vi "Regatron.G5.Rest Simple Example.vi"() -> ()   [LabVIEW 2021, in "G5 Regatron Custom Device Shared.lvlib"]
doc: "Simple Example to control a G5 device"
uses:
  G5 Regatron Custom Device/Shared/G5 Regatron Custom Device Shared.lvlib
  Regatron.G5.Rest System.llb/G5.Rest System Output References.ctl
  Regatron.G5.Rest System.llb/G5.Rest System Output Limits.ctl
  Regatron.G5.Rest System.llb/G5.Rest System Output Values.ctl
  Regatron.G5.Rest Handle.llb/G5.Rest Status.ctl
  Regatron.G5.Rest System.llb/G5.Rest System Output Limits Datasource.ctl
  Regatron.G5.Rest System.llb/G5.Rest System Output References Datasource.ctl
  Regatron.G5.Rest System.llb/G5.Rest System Clear Inicidents.ctl
  Regatron.G5.Rest.lvlib
panel:
  in  "Registerkartenelement":enum32{"Power", "Limits"}(tab)
  in  "SET Output Control":T1(ring)
  out "Output Values":T2 {"Power W" format="%#.2f"; "Load R Ohm" format="%#_3e"; "Power kW" format="%#_3e"; "Current A" format="%#.2f"; "Voltage V" format="%#.2f"}
  in  "Clear Error & Warnings":bool
  out "State":T3(ring)=enum."Ready"
  in  "Power OFF/ON":bool
  in  "SET Output Reference":T4 {"Load R Ohm" format="%#_3e"; "Power W" format="%#.2f"; "Current A" format="%#.2f"; "Voltage V" format="%#.2f"}
  out "Device found":bool
  out "System Device":i32
  in  "SET Output Limit":T5 {"Power Lower Limit W" format="%#.2f"; "Power Upper Limit W" format="%#.2f"; "Current Lower Limit A" format="%#.2f"; "Current Upper Limit A" format="%#.2f"; "Voltage Lower Limit V" format="%#.2f"; "Voltage Upper Limit V" format="%#.2f"}
  in  "Stopp-Schaltfläche":bool
  out "Error Out":errorcluster
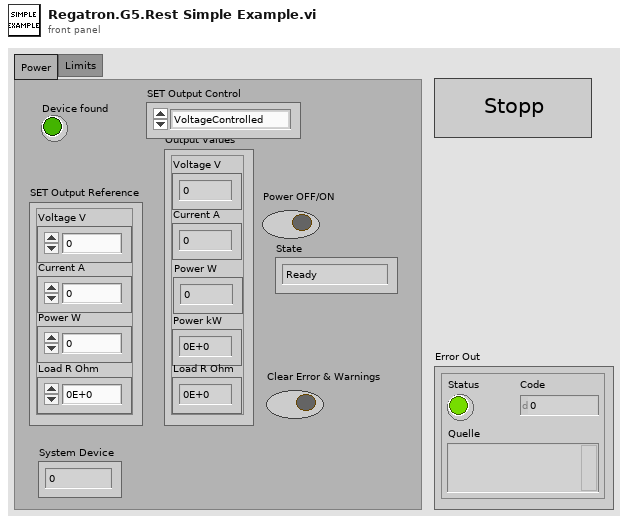
[diagram p1: front panel]
types:
  T1 = enum16{"VoltageControlled", "CurrentControlled", "PowerControlled", "ResistanceControlled"}
  T2 = typedef "G5 Regatron Custom Device Shared.lvlib/Regatron.G5.Rest.lvlib/G5.Rest System Output Values.ctl" = cluster{"Voltage V":sgl, "Current A":sgl, "Power W":sgl, "Power kW":sgl, "Load R Ohm":sgl}
  T3 = enum16{"Undefined", "PowerUp", "NotReady", "Ready", "VoltageOnPrepare", "VoltageOn", "VoltageOnLeave", "Test", "FirmwareUpdate"}
  T4 = typedef "G5 Regatron Custom Device Shared.lvlib/Regatron.G5.Rest.lvlib/G5.Rest System Output References.ctl" = cluster{"Voltage V":sgl, "Current A":sgl, "Power W":sgl, "Load R Ohm":sgl}
  T5 = typedef "G5 Regatron Custom Device Shared.lvlib/Regatron.G5.Rest.lvlib/G5.Rest System Output Limits.ctl" = cluster{"Voltage Upper Limit V":sgl, "Voltage Lower Limit V":sgl, "Current Upper Limit A":sgl, "Current Lower Limit A":sgl, "Power Upper Limit W":sgl, "Power Lower Limit W":sgl}
  T6 = typedef "G5 Regatron Custom Device Shared.lvlib/Regatron.G5.Rest.lvlib/G5.Rest Status.ctl" = enum16{"Read", "Write"}
  T7 = typedef "G5 Regatron Custom Device Shared.lvlib/Regatron.G5.Rest.lvlib/G5.Rest System Clear Inicidents.ctl" = enum16{"Clear Errors and Warnings", "Clear Warnings", "Clear Errors"}
  T8 = typedef "G5 Regatron Custom Device Shared.lvlib/Regatron.G5.Rest.lvlib/G5.Rest System Output References Datasource.ctl" = enum16{"Voltage", "Current", "Power", "Load Resistance", "ALL"}[]
  T9 = typedef "G5 Regatron Custom Device Shared.lvlib/Regatron.G5.Rest.lvlib/G5.Rest System Output Limits Datasource.ctl" = enum16{"Voltage Upper Limit", "Voltage Lower Limit", "Current Upper Limit", "Current Lower Limit", "Power Upper Limit", "Power Lower Limit", "ALL"}[]
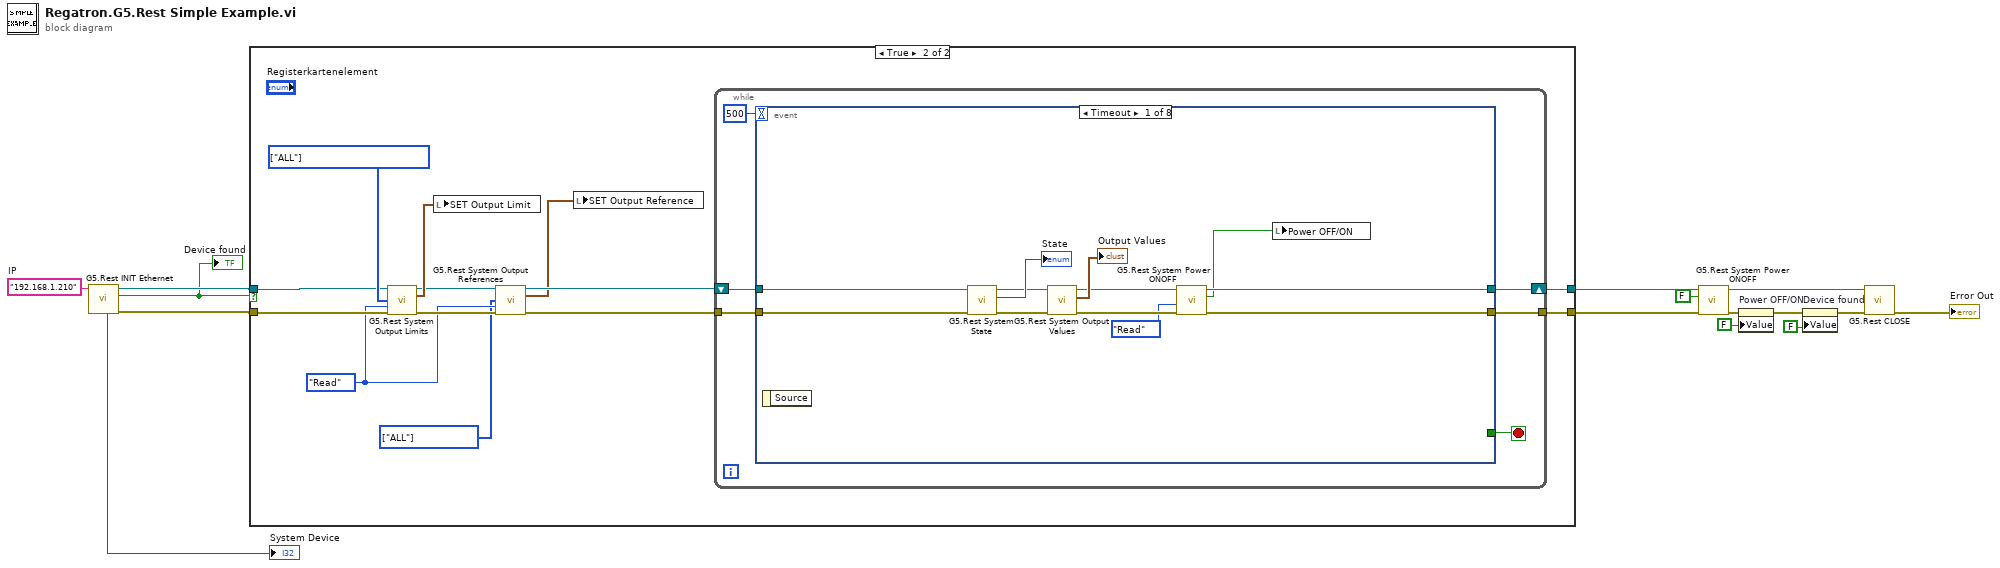
[diagram p0: block diagram]
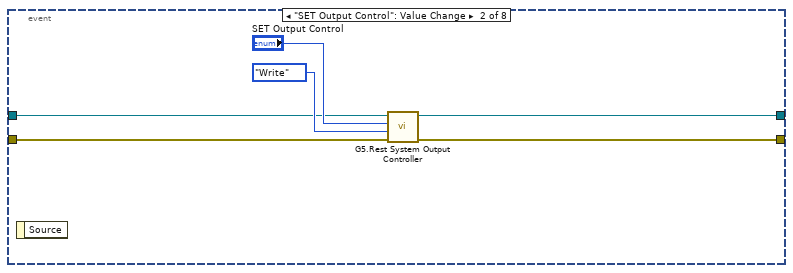
[diagram p3: hidden frame]
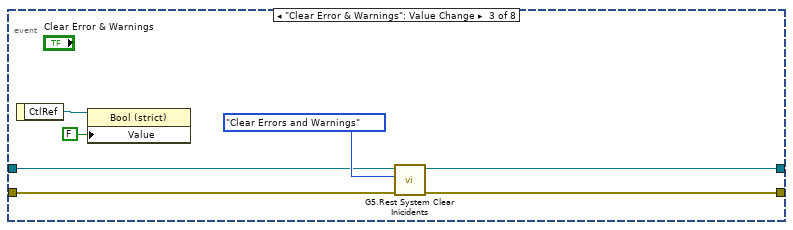
[diagram p4: hidden frame]
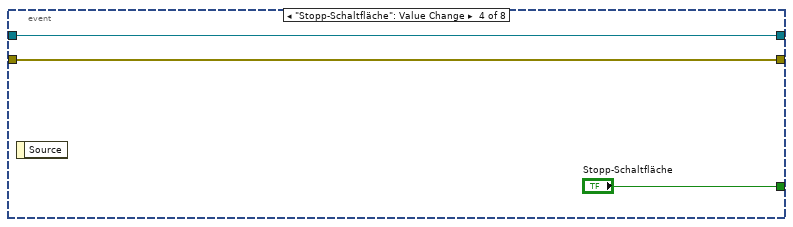
[diagram p5: hidden frame]
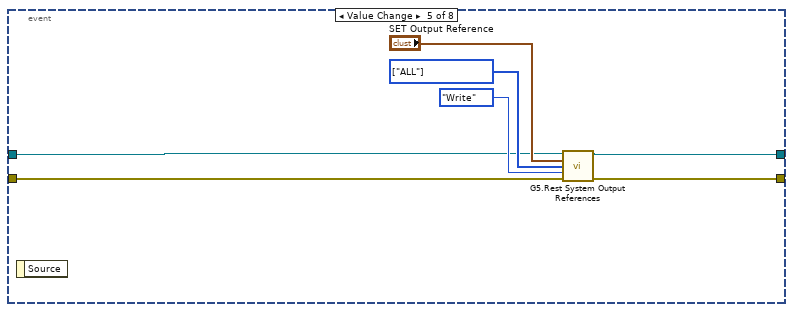
[diagram p6: hidden frame]
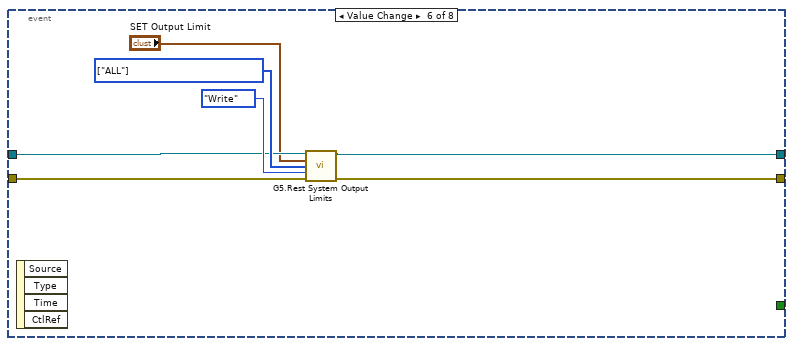
[diagram p7: hidden frame]
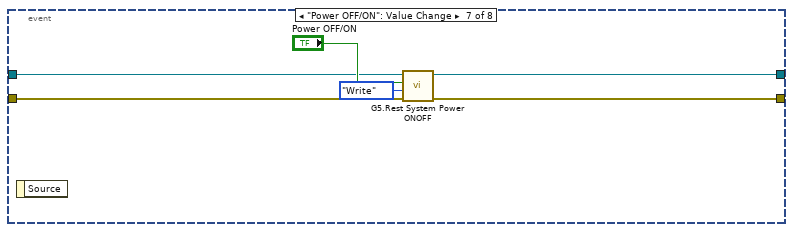
[diagram p8: hidden frame]
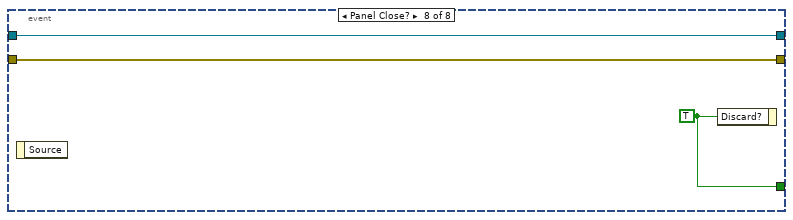
[diagram p9: hidden frame]
diagram:
  w5 = "192.168.1.210"  # IP
  n1 = call "G5.Rest INIT Ethernet.vi"("IP"=w5) -> ("error out"=w4:errorcluster, "Device found"=w2:bool, "G5 WEB API"=w3:refnum<class "REST Client.lvclass">, "Modul size"=→"System Device":i32)  [unwired: 6 in, 1 out]
  "Device found" <- w2
  n2 = case shown="True" w2 {
    tunnel: w4 -> [w17 w27]
    tunnel: [w17 w30] -> w9
    tunnel: [w16 w29] -> w7
    tunnel: w3 -> [w16 w19]
    frame False {
    }
    frame True {
      w20 = T8 [enum."ALL"] items=["Voltage", "Current", "Power", "Load Resistance", "ALL"] ("Datasource")
      w21 = T9 [enum."ALL"] items=["Voltage Upper Limit", "Voltage Lower Limit", "Current Upper Limit", "Current Lower Limit", "Power Upper Limit", "Power Lower Limit", "ALL"] ("Datasource")
      w22 = G5.Rest_Status."Read" ("Status")
      n3 = call "G5.Rest System Output Limits.vi"("G5 WEB API (Eingang)"=w19, "Datasource"=w21, "Status"=w22, "Fehler (Eingang, kein Fehler)"=w27) -> ("G5 WEB API (Ausgang)"=w18:refnum<class "REST Client.lvclass">, "GET Output Limit"=w24:T5, "Fehler (Ausgang)"=w26:errorcluster)  [unwired: 9 in]
      n4 = local write "SET Output Limit"(w24) -> ()
      n5 = call "G5.Rest System Output References .vi"("G5 WEB API (Eingang)"=w18, "Datasource"=w20, "Status"=w22, "Fehler (Eingang, kein Fehler)"=w26) -> ("G5 WEB API (Ausgang)"=w25:refnum<class "REST Client.lvclass">, "GET Output Reference"=w23:T4, "Fehler (Ausgang)"=w28:errorcluster)  [unwired: 9 in]
      n6 = local write "SET Output Reference"(w23) -> ()
      n7 = while {
        tunnel: w28 -> [w34]
        tunnel: [w33] -> w30
        shift-right: [w32] -> w29
        shift-left: w25 -> [w31]
        stop <- w35 stop-if-true
        n8 = event shown="[0] Timeout" {
          selector: _ -> [_ _ _ _ _ _ _ _]
          dyn-events: _ -> [_ _ _ _ _ _ _ _]
          timeout: 500 -> [_ _ _ _ _ _ _ _]
          tunnel: [_ _ _ "Stopp-Schaltfläche" _ _ _ w87] -> w35
          tunnel: w34 -> [w37 w54 w61 w63 w65 w78 w83 w86]
          tunnel: [w44 w53 w60 w63 w70 w74 w82 w86] -> w33
          tunnel: [w43 w49 w55 w62 w67 w73 w81 w85] -> w32
          tunnel: w31 -> [w38 w50 w56 w62 w66 w75 w80 w85]
          event Timeout {
            n9 = event-data() -> ()  [unwired: 1 in, 1 out]
            n10 = call "G5.Rest System State.vi"("Fehler (Eingang, kein Fehler)"=w37, "G5 WEB API (Eingang)"=w38) -> ("Fehler (Ausgang)"=w40:errorcluster, "GET State"=→"State":T3, "G5 WEB API (Ausgang)"=w46:refnum<class "REST Client.lvclass">)  [unwired: 7 in]
            n11 = call "G5.Rest System Output Values.vi"("Fehler (Eingang, kein Fehler)"=w40, "G5 WEB API (Eingang)"=w46) -> ("Fehler (Ausgang)"=w45:errorcluster, "Output Values"=→"Output Values":T2, "G5 WEB API (Ausgang)"=w39:refnum<class "REST Client.lvclass">)  [unwired: 7 in]
            n12 = call "G5.Rest System Power ONOFF.vi"("Fehler (Eingang, kein Fehler)"=w45, "Status"=G5.Rest_Status."Read", "G5 WEB API (Eingang)"=w39) -> ("Fehler (Ausgang)"=w44:errorcluster, "Get Power OFF/ON"=w41:bool, "G5 WEB API (Ausgang)"=w43:refnum<class "REST Client.lvclass">)  [unwired: 6 in]
            n13 = local write "Power OFF/ON"(w41) -> ()
          }
          event "SET Output Control": Value Change {
            n14 = event-data() -> ()  [unwired: 1 in, 1 out]
            n15 = call "G5.Rest System Output Controller.vi"("Fehler (Eingang, kein Fehler)"=w54, "Status"=G5.Rest_Status."Write", "SET Output Control"="SET Output Control", "G5 WEB API (Eingang)"=w50) -> ("Fehler (Ausgang)"=w53:errorcluster, "G5 WEB API (Ausgang)"=w49:refnum<class "REST Client.lvclass">)  [unwired: 5 in, 1 out]
          }
          event "Clear Error & Warnings": Value Change {
            n16 = event-data() -> ("CtlRef"=w58:refnum<vi>)  [unwired: 1 in]
            n17 = property class="Bool (strict)"(reference=w58, "Value"=FALSE ("Wert")) -> ()  [unwired: 1 in, 2 out]
            n18 = call "G5.Rest System Clear Inicidents.vi"("Fehler (Eingang, kein Fehler)"=w61, "Clear Inicidents"=G5.Rest_System_Clear_Inicidents."Clear Errors and Warnings", "G5 WEB API (Eingang)"=w56) -> ("Fehler (Ausgang)"=w60:errorcluster, "G5 WEB API (Ausgang)"=w55:refnum<class "REST Client.lvclass">)  [unwired: 7 in]
          }
          event "Stopp-Schaltfläche": Value Change {
            n19 = event-data() -> ()  [unwired: 1 in, 1 out]
          }
          event Value Change {
            w69 = T8 [enum."ALL"] items=["Voltage", "Current", "Power", "Load Resistance", "ALL"] ("Datasource")
            n20 = event-data() -> ()  [unwired: 1 in, 1 out]
            n21 = call "G5.Rest System Output References .vi"("G5 WEB API (Eingang)"=w66, "SET Output Reference"="SET Output Reference", "Datasource"=w69, "Status"=G5.Rest_Status."Write", "Fehler (Eingang, kein Fehler)"=w65) -> ("G5 WEB API (Ausgang)"=w67:refnum<class "REST Client.lvclass">, "Fehler (Ausgang)"=w70:errorcluster)  [unwired: 8 in, 1 out]
          }
          event Value Change {
            w77 = T9 [enum."ALL"] items=["Voltage Upper Limit", "Voltage Lower Limit", "Current Upper Limit", "Current Lower Limit", "Power Upper Limit", "Power Lower Limit", "ALL"] ("Datasource")
            n22 = event-data() -> ()  [unwired: 1 in, 4 out]
            n23 = call "G5.Rest System Output Limits.vi"("G5 WEB API (Eingang)"=w75, "SET Output Limit"="SET Output Limit", "Datasource"=w77, "Status"=G5.Rest_Status."Write", "Fehler (Eingang, kein Fehler)"=w78) -> ("G5 WEB API (Ausgang)"=w73:refnum<class "REST Client.lvclass">, "Fehler (Ausgang)"=w74:errorcluster)  [unwired: 8 in, 1 out]
          }
          event "Power OFF/ON": Value Change {
            n24 = event-data() -> ()  [unwired: 1 in, 1 out]
            n25 = call "G5.Rest System Power ONOFF.vi"("Fehler (Eingang, kein Fehler)"=w83, "Status"=G5.Rest_Status."Write", "Power OFF/ON"="Power OFF/ON", "G5 WEB API (Eingang)"=w80) -> ("Fehler (Ausgang)"=w82:errorcluster, "G5 WEB API (Ausgang)"=w81:refnum<class "REST Client.lvclass">)  [unwired: 5 in, 1 out]
          }
          event Panel Close? {
            w87 = TRUE ("Verwerfen?")
            n26 = event-data() -> ()  [unwired: 1 in, 1 out]
            n27 = event-data("Discard?"=w87) -> ()  [unwired: 1 in, 1 out]
          }
        }
      }
    }
  }
  n28 = call "G5.Rest System Power ONOFF.vi"("Fehler (Eingang, kein Fehler)"=w9, "Power OFF/ON"=FALSE, "G5 WEB API (Eingang)"=w7) -> ("Fehler (Ausgang)"=w14:errorcluster, "G5 WEB API (Ausgang)"=w6:refnum<class "REST Client.lvclass">)  [unwired: 6 in, 1 out]
  n29 = property on="Power OFF/ON" class="Bool (strict)"(error in=w14, "Value"=FALSE ("Power OFF/ON")) -> (error out=w12:errorcluster)  [unwired: 1 in, 1 out]
  n30 = property on="Device found" class="Bool (strict)"(error in=w12, "Value"=FALSE ("Device found")) -> (error out=w11:errorcluster)  [unwired: 1 in, 1 out]
  n31 = call "G5.Rest CLOSE.vi"("Fehler (Eingang, kein Fehler)"=w11, "G5 WEB API"=w6) -> ("error out"=→"Error Out":errorcluster)  [unwired: 9 in]
